vi "1D boolean to digital.vi"() -> ()   [LabVIEW 2010]
uses:
  <vilib>/Waveform/DTblOps.llb/DTbl Boolean Array to Digital.vi
panel:
  in  "Array":bool[](array[boolean])
  out "Digital Waveform Graph":digitalwaveform(graph)
  # "This example demonstrates how to convert a 1D array of booleans with any number of elements\n into a Digital Waveform. By using a for loop it would be possible to modify the code to take\na 2D array of booleans and convert it into a 2D array of Digital Waveforms.\nThis is particularly useful for generating patterns to use with DAQmx Digital Outputs."
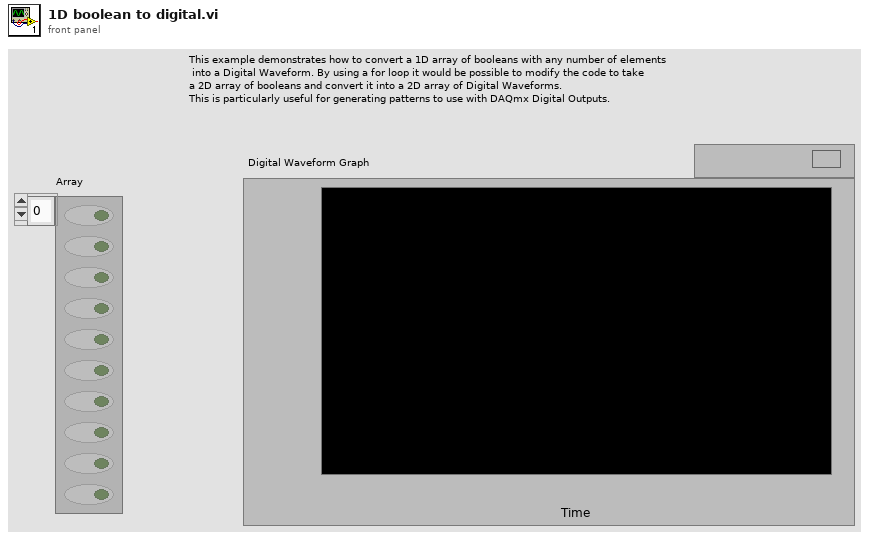
[diagram p1: front panel]
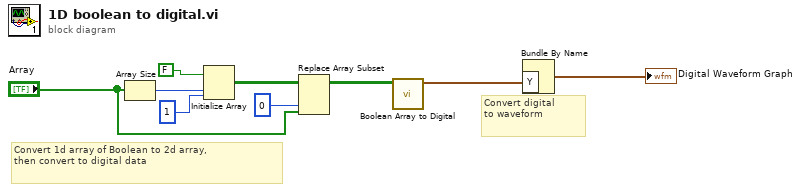
[diagram p0: block diagram]
diagram:
  # "Convert digital\nto waveform"
  # "Convert 1d array of Boolean to 2d array,\nthen convert to digital data"
  n1 = Array Size(array="Array") -> (size(s)=w6:i32)
  n2 = Initialize Array(FALSE, w6, 1 ("dimension size")) -> (w5:bool[][])
  n3 = Replace Array Subset(array=w5, new element="Array", index (col)=0 ("index (row)")) -> (w8:bool[][])  [unwired: 1 in]
  n4 = call-poly <vilib>:"Boolean Array to Digital.vi"("boolean array"=w8) -> ("digital data"=w7:digitaldata)  [unwired: 3 in, 7 out]
  n5 = Bundle By Name("Y"=w7) -> (→"Digital Waveform Graph":digitalwaveform)  [unwired: 1 in]
